vi "general_measurement_KT_3.vi"(9 "Data Keithley":dbl[](array[numeric]), 10 "Array 4":dbl[](array[numeric]), 11 "Array 3":dbl[](array[numeric])) -> (2 "Array":dbl[](array[numeric]), 3 "Array 2":dbl[](array[numeric]), 4 "Data Out":dbl[](array[numeric]), 5 "Seebeck coefficient":cluster{"Y":dbl[], "Y":dbl[]}[](graph))   [LabVIEW 2011]
uses:
  <vilib>/express/express arith-compare/Formula/XNode/ExpressFormulaBlockNode.xnode
panel:
  in  "Current":bool=TRUE
  out "Array Time Out":dbl[][](array[numeric])
  out "Array Temp Out":dbl[][](array[numeric])
  in  "Array Time In":dbl[][](array[numeric])
  in  "Array Temp In":dbl[][](array[numeric])
  out "Temp Graph":cluster{"Y":dbl[], "Y":dbl[]}[](graph)
  in  "General Time":dbl
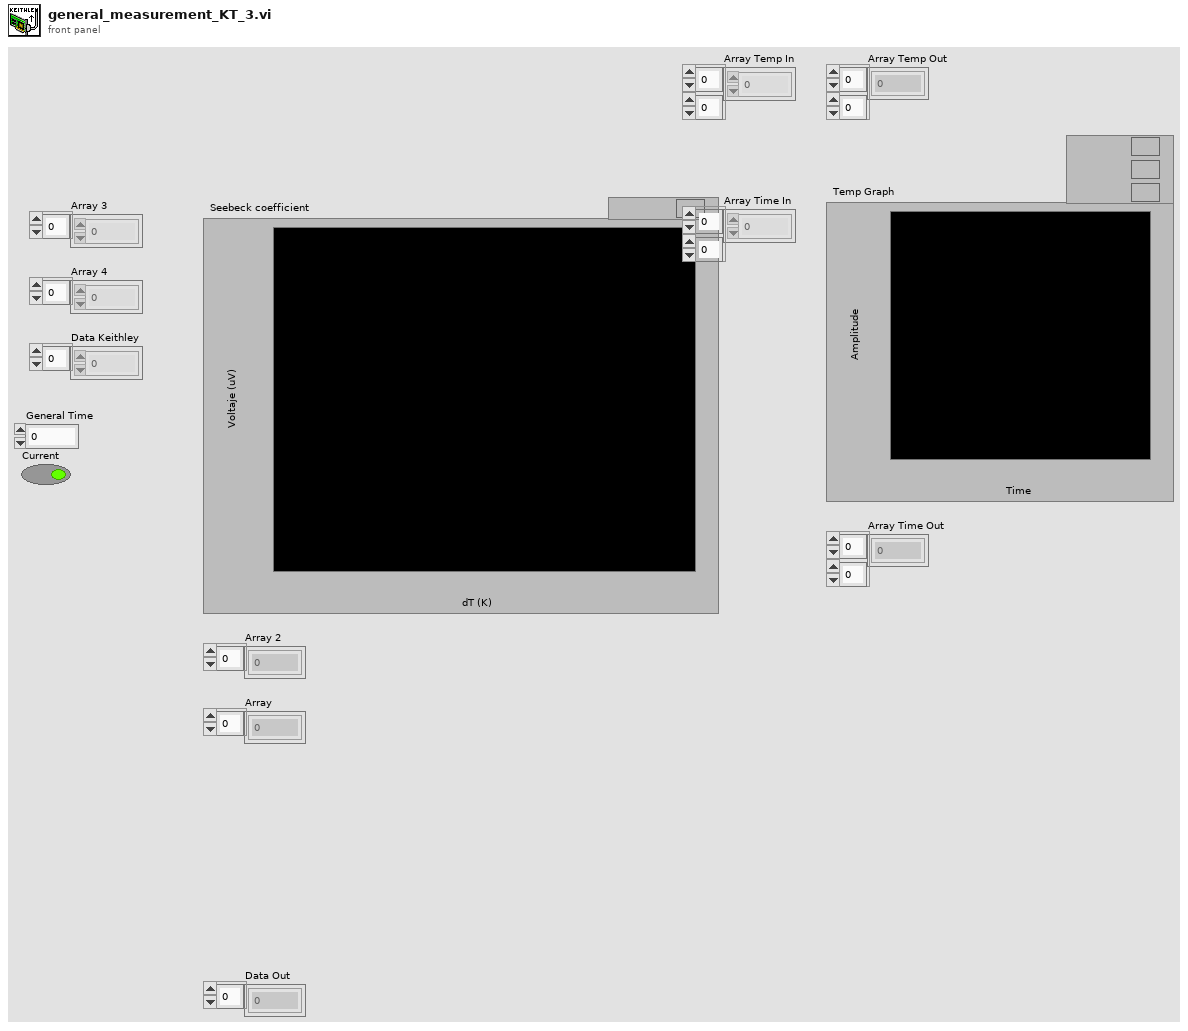
[diagram p1: front panel]
types:
  T1 = cluster{"Data Keithley[0]":dbl, "Data Keithley[1]":dbl, "Data Keithley[2]":dbl, "Data Keithley[3]":dbl, "Data Keithley[4]":dbl, "Data Keithley[5]":dbl, "Data Keithley[6]":dbl, "Data Keithley[7]":dbl, "Data Keithley[8]":dbl}
  T2 = cluster{"[0]":dbl, "[1]":dbl, "[2]":dbl, "[3]":dbl, "[4]":dbl, "[5]":dbl, "[6]":dbl, "[7]":dbl, "[8]":dbl}
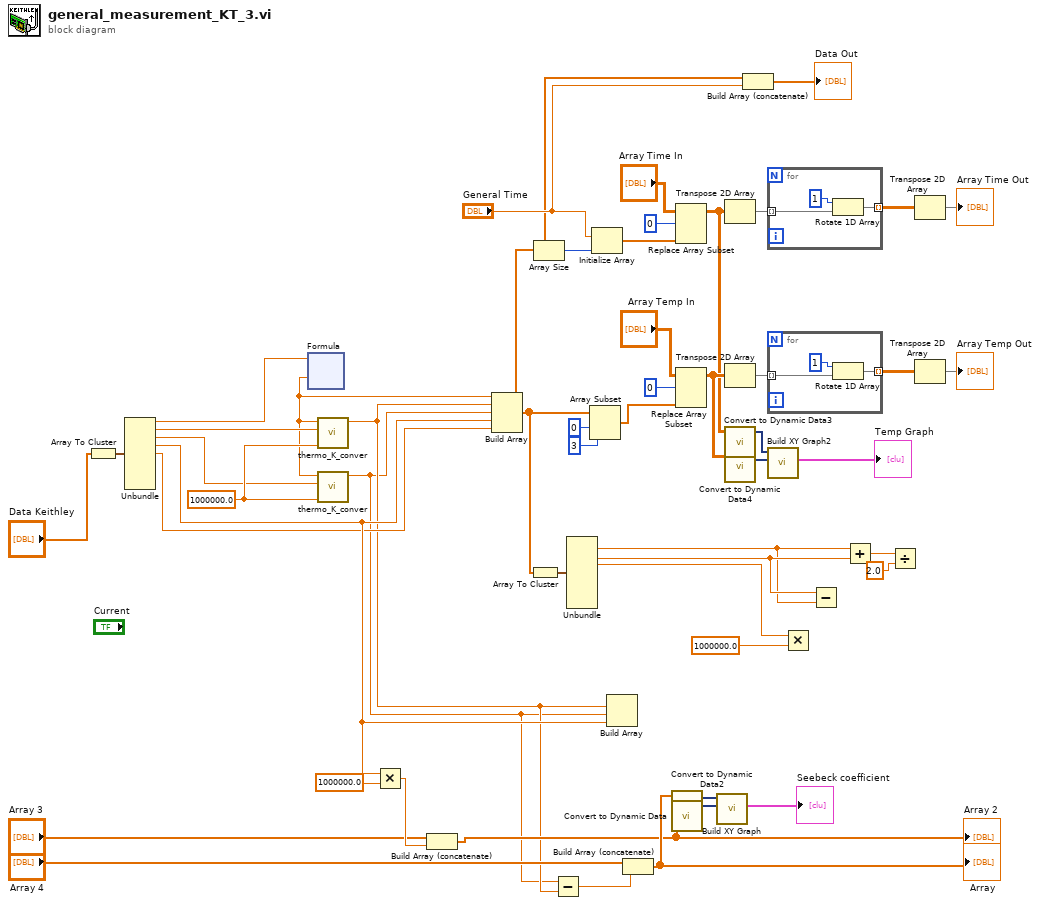
[diagram p0: block diagram]
diagram:
  w39 = 1000000.0 ("y")
  n1 = Array To Cluster(array="Data Keithley") -> (cluster=w41:T1)
  n2 = Unbundle(w41) -> ("Data Keithley[0]"=w38:dbl, "Data Keithley[1]"=w37:dbl, "Data Keithley[2]"=w36:dbl, "Data Keithley[3]"=w17:dbl, "Data Keithley[4]"=w16:dbl)  [unwired: 4 out]
  n3 = xnode ("Formula")("R"=w38) -> ("Result"=w35:dbl)  [unwired: 1 in, 1 out]
  n4 = call "thermo_K_conver.vi"("y"=w39, "Measurement Data[1]"=w37, "Measurement Data[0]"=w35) -> ("Result"=w10:dbl)  [unwired: 8 in]
  n5 = call "thermo_K_conver.vi"("y"=w39, "Measurement Data[1]"=w36, "Measurement Data[0]"=w35) -> ("Result"=w9:dbl)  [unwired: 8 in]
  n6 = Multiply(x=w17, y=1000000.0 ("x")) -> (x*y=w51:dbl)
  n7 = Build Array (concatenate)("Array 3", w51) -> (w47:dbl[])
  "Array 2" <- w47
  n8 = Build Array(w35, w10, w9, w17, w16) -> (w5:dbl[])
  n9 = Array To Cluster(array=w5) -> (cluster=w6:T2)
  n10 = Array Size(array=w5) -> (size(s)=w21:i32)
  n11 = Subtract(x=w9, y=w10) -> (x-y=w45:dbl)
  n12 = Unbundle(w6) -> ("[1]"=w3:dbl, "[2]"=w4:dbl, "[3]"=w2:dbl)  [unwired: 6 out]
  n13 = Array Subset(array=w5, index=0, length=3) -> (w13:dbl[])
  n14 = Initialize Array("General Time", w21) -> (w20:dbl[])
  n15 = Build Array(w10, w9, w17) -> ()  [unwired: 1 in, 1 out]
  n16 = Build Array (concatenate)("Array 4", w45) -> (w49:dbl[])
  "Array" <- w49
  n17 = call "Convert to Dynamic Data2"("Array"=w49) -> ("Dynamic Data Type"=w50:dynamicdata)  [unwired: 3 in]
  n18 = call "Convert to Dynamic Data"("Array"=w47) -> ("Dynamic Data Type"=w48:dynamicdata)  [unwired: 3 in]
  n19 = Replace Array Subset(array="Array Time In", new element=w20, index (row)=0) -> (w30:dbl[][])  [unwired: 1 in]
  n20 = Replace Array Subset(array="Array Temp In", new element=w13, index (row)=0) -> (w32:dbl[][])  [unwired: 1 in]
  n21 = call "Build XY Graph"("Y Input"=w48, "X Input"=w50) -> ("XY Graph"=→"Seebeck coefficient":cluster{"Y":dbl[], "Y":dbl[]}[])  [unwired: 3 in, 6 out]
  n22 = Transpose 2D Array(2D array=w30) -> (transposed array=w23:dbl[][])
  n23 = Transpose 2D Array(2D array=w32) -> (transposed array=w26:dbl[][])
  n24 = call "Convert to Dynamic Data3"("2D Array"=w30) -> ("Dynamic Data Type"=w18:dynamicdata)  [unwired: 3 in]
  n25 = call "Convert to Dynamic Data4"("2D Array"=w32) -> ("Dynamic Data Type"=w19:dynamicdata)  [unwired: 3 in]
  n26 = Build Array (concatenate)(w5, "General Time") -> (→"Data Out":dbl[])
  n27 = for {
    tunnel: w23 -> [w54] mode=indexing
    tunnel: [w53] -> w24 mode=indexing
    n28 = Rotate 1D Array(1:w54, 2:1 ("n")) -> (0:w53:dbl[])
  }
  n29 = for {
    tunnel: w26 -> [w57] mode=indexing
    tunnel: [w56] -> w27 mode=indexing
    n30 = Rotate 1D Array(1:w57, 2:1 ("n")) -> (0:w56:dbl[])
  }
  n31 = call "Build XY Graph2"("Y Input"=w19, "X Input"=w18) -> ("XY Graph"=→"Temp Graph":cluster{"Y":dbl[], "Y":dbl[]}[])  [unwired: 3 in, 6 out]
  n32 = Multiply(x=w2, y=1000000.0 ("x")) -> ()  [unwired: 1 out]
  n33 = Subtract(x=w4, y=w3) -> ()  [unwired: 1 out]
  n34 = Add(x=w3, y=w4) -> (x+y=w8:dbl)
  n35 = Divide(x=w8, y=2.0) -> ()  [unwired: 1 out]
  n36 = Transpose 2D Array(2D array=w24) -> (transposed array=→"Array Time Out":dbl[][])
  n37 = Transpose 2D Array(2D array=w27) -> (transposed array=→"Array Temp Out":dbl[][])
